vi "Set IPS Switch Heater.vi"(8 "error in (no error)":errorcluster, 10 "Switch Heater Status":T1, 11 "Instrument.Oxford1820 in":refnum<class "Instrument.OxfordVRM.lvclass">) -> (0 "error out":errorcluster, 2 "Response":string, 3 "Instrument.Oxford1820 out":refnum<class "Instrument.OxfordVRM.lvclass">)   [LabVIEW 2016, in "Instrument.OxfordVRM.lvclass"]
uses:
  Instrument.OxfordVRM.lvclass
  <instrlib>/Mercury iXX/Public/Libraries/Magnet/Controls/Switch Heater.ctl
  Instrument.OxfordVRM.lvclass/Instrument.OxfordVRM.ctl
  <instrlib>/Mercury iXX/Public/Controls/Response String.ctl
  <instrlib>/Mercury iXX/Public/Libraries/Magnet/Open/Open Magnet Device.vi
  <instrlib>/Mercury iXX/Public/Libraries/Magnet/Signals/Read/Current (Read).vi
  <instrlib>/Mercury iXX/Public/Libraries/Magnet/Signals/Read/Persistant Current (Read).vi
  <instrlib>/Mercury iXX/Public/Libraries/Magnet/Signals/Set/Switch Heater Status (Set).vi
  <instrlib>/Mercury iXX/Public/Libraries/Magnet/Signals/Read/Switch Heater Status (Read).vi
  <instrlib>/Mercury iXX/Mercury iXX.lvlib
  <instrlib>/Mercury iXX/Public/Libraries/Magnet.lvlib
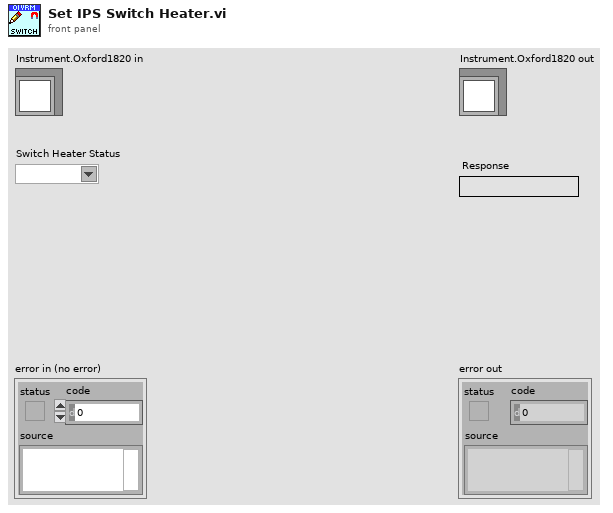
[diagram p1: front panel]
types:
  T1 = typedef "Mercury iXX.lvlib/Magnet.lvlib/Switch Heater.ctl" = string
  T2 = typedef "Mercury iXX.lvlib/Response String.ctl" = string
  T3 = typedef "Mercury iXX.lvlib/Mercury Reference.ctl" = cluster{"Comms":refnum<visa-resource-name>, "Device ID":string[], "Comms Layer":T4, "Command":string, "Query reference":T5}
  T4 = typedef "Mercury iXX.lvlib/Comms Transport Layer.ctl" = enum16{"Ethernet TCP/IP", "USB", "ISOBus - RS-232", "GPIB"}
  T5 = typedef "Mercury iXX.lvlib/Query Dynamic Reference.ctl" = refnum<vi>
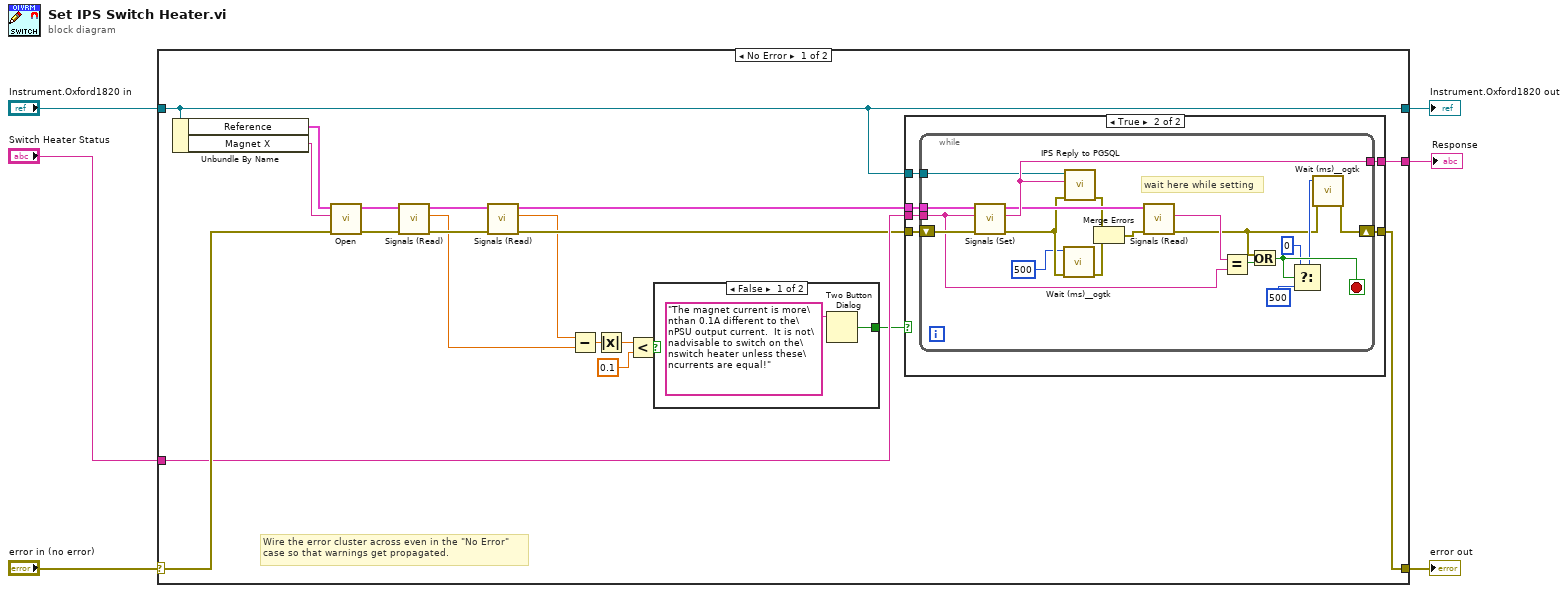
[diagram p0: block diagram]
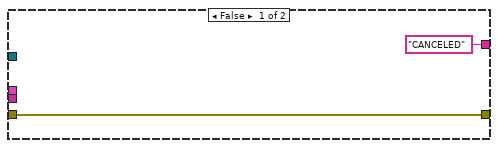
[diagram p2: hidden frame]
diagram:
  n1 = case shown="No Error" "error in (no error)" {
    selector: "error in (no error)" -> [w13 w58]
    tunnel: [w26 w58] -> w5
    tunnel: [w24 w57] -> w3
    tunnel: "Instrument.Oxford1820 in" -> [w24 w57]
    tunnel: [w25 _] -> w2
    tunnel: "Switch Heater Status" -> [w12 _]
    frame No Error {
      # "Wire the error cluster across even in the \"No Error\"\ncase so that warnings get propagated."
      n2 = Unbundle By Name(w24) -> ("Reference"=w23:T3, "Magnet X"=w22:string)
      n3 = call-poly <instrlib>:"Open.vi"("error in (no error)"=w13, "Device Identifier"=w22, "Mercury Reference In"=w23) -> ("error out"=w16:errorcluster, "Mercury Reference Out"=w15:T3)  [unwired: 7 out]
      n4 = call-poly <instrlib>:"Signals (Read).vi"("error in"=w16, "Mercury Reference In"=w15) -> ("error out"=w18:errorcluster, "Current"=w8:dbl, "Mercury Reference Out"=w17:T3)  [unwired: 1 in, 6 out]
      n5 = call-poly <instrlib>:"Signals (Read).vi"("error in"=w18, "Mercury Reference In"=w17) -> ("error out"=w11:errorcluster, "Persistant Current"=w9:dbl, "Mercury Reference Out"=w10:T3)  [unwired: 1 in, 6 out]
      n6 = Subtract(x=w9, y=w8) -> (x-y=w19:dbl)
      n7 = Absolute Value(x=w19) -> (abs(x)=w20:dbl)
      n8 = Less?(x=w20, y=0.1) -> (x < y?=w21:bool)
      n9 = case shown="False" w21 {
        selector: w21 -> [_ w56]
        tunnel: [w55 w56] -> w7
        frame False {
          n10 = Two Button Dialog(message="The magnet current is more\nthan 0.1A different to the\nPSU output current.  It is not\nadvisable to switch on the\nswitch heater unless these\ncurrents are equal!") -> (T button?=w55:bool)  [unwired: 2 out]
        }
        frame True {
        }
      }
      n11 = case shown="True" w7 {
        tunnel: [w28 w34] -> w26
        tunnel: [T2 "CANCELED" ("Response") w33] -> w25
        tunnel: w24 -> [_ w32]
        tunnel: w12 -> [_ w31]
        tunnel: w11 -> [w28 w30]
        tunnel: w10 -> [_ w29]
        frame False {
        }
        frame True {
          n12 = while {
            tunnel: [w53] -> w33
            tunnel: w32 -> [w52]
            tunnel: w31 -> [w46]
            tunnel: w29 -> [w47]
            shift-right: [w41] -> w34
            shift-left: w30 -> [w48]
            stop <- w45 stop-if-true
            # "wait here while setting"
            n13 = call-poly <instrlib>:"Signals (Set).vi"("error in"=w48, "Switch Heater Status"=w46, "Mercury Reference In"=w47) -> ("error out"=w39:errorcluster, "Response"=w53:T2, "Mercury Reference Out"=w51:T3)  [unwired: 1 in, 5 out]
            n14 = call <userlib>:"Wait (ms)__ogtk.vi"("error in (no error)"=w39, "milliseconds to wait"=u32 500) -> ("error out"=w35:errorcluster)  [unwired: 8 in, 1 out]
            n15 = call "IPS Reply to PGSQL.vi"("error in (no error)"=w39, "Response"=w53, "Instrument.1820 in"=w52) -> ("error out"=w37:errorcluster)  [unwired: 7 in, 1 out]
            n16 = Merge Errors(w37, w35) -> (w36:errorcluster)
            n17 = call-poly <instrlib>:"Signals (Read).vi"("error in"=w36, "Mercury Reference In"=w51) -> ("error out"=w40:errorcluster, "Switch Heater Status"=w50:string)  [unwired: 1 in, 7 out]
            n18 = Equal?(x=w50, y=w46) -> (x = y?=w49:bool)
            n19 = Or(x=w40, y=w49) -> (x .or. y?=w45:bool)
            n20 = Select(t=u32 0, s=w45, f=u32 500 ("milliseconds to wait")) -> (s? t:f=w42:u32)
            n21 = call <userlib>:"Wait (ms)__ogtk.vi"("error in (no error)"=w40, "milliseconds to wait"=w42) -> ("error out"=w41:errorcluster)  [unwired: 8 in, 1 out]
          }
        }
      }
    }
    frame Error {
    }
  }
  "error out" <- w5
  "Instrument.Oxford1820 out" <- w3
  "Response" <- w2
